vi "Sets the Value for the MX+B Function.vi"(5 "Enable to Query":bool=TRUE, 7 "Enable to Sets":bool=TRUE, 8 "error in":errorcluster, 9 "Offset Factor B":dbl, 10 "Scale Factor M":dbl, 11 "VISA resource name":refnum<visa-resource-name>) -> (0 "error out":errorcluster, 1 "Return the Offset Factor B":string, 2 "Return the Scale Factor M":string, 3 "VISA resource name out":refnum<visa-resource-name>)   [LabVIEW 2011, in "DMM4.lvlib"]
uses:
  <instrlib>/DMM4/DMM4.lvlib
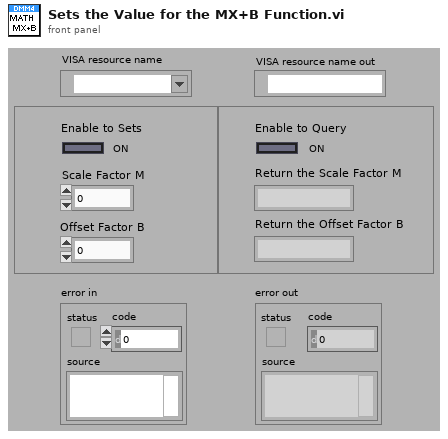
[diagram p1: front panel]
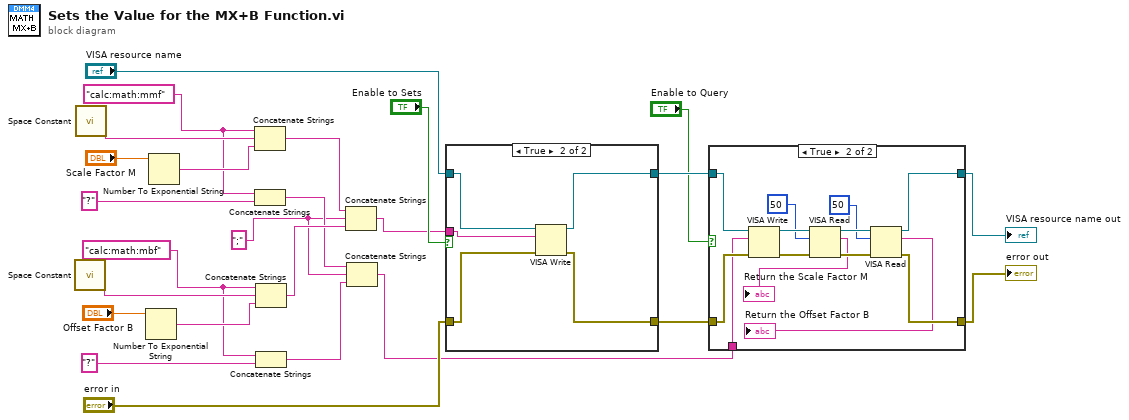
[diagram p0: block diagram]
diagram:
  w12 = ";"
  w16 = "calc:math:mbf"
  w17 = "calc:math:mmf"
  n1 = call <vilib>:"Space Constant.vi"() -> ("String"=w20:string)
  n2 = call <vilib>:"Space Constant.vi"() -> ("String"=w22:string)
  n3 = Number To Exponential String(number="Offset Factor B") -> (E-format string=w21:string)  [unwired: 3 in]
  n4 = Number To Exponential String(number="Scale Factor M") -> (E-format string=w23:string)  [unwired: 3 in]
  n5 = Concatenate Strings(w17, w22, w23) -> (w15:string)
  n6 = Concatenate Strings(w17, "?") -> (w13:string)
  n7 = Concatenate Strings(w16, w20, w21) -> (w14:string)
  n8 = Concatenate Strings(w16, "?") -> (w11:string)
  n9 = Concatenate Strings(w15, w12, w14) -> (w7:string)
  n10 = Concatenate Strings(w13, w12, w11) -> (w1:string)
  n11 = case shown="True" "Enable to Sets" {
    tunnel: "VISA resource name" -> [w27 w32]
    tunnel: "error in" -> [w26 w31]
    tunnel: [w27 w30] -> w6
    tunnel: [w26 w29] -> w5
    tunnel: w7 -> [_ w28]
    frame False {
    }
    frame True {
      n12 = VISA Write(VISA resource name=w32, write buffer=w28, error in (no error)=w31) -> (VISA resource name out=w30:refnum<visa-resource-name>, error out=w29:errorcluster)  [unwired: 1 out]
    }
  }
  n13 = case shown="True" "Enable to Query" {
    tunnel: w6 -> [w34 w41]
    tunnel: w5 -> [w33 w40]
    tunnel: [w34 w39] -> w4
    tunnel: [w33 w38] -> w3
    tunnel: w1 -> [_ w35]
    frame False {
    }
    frame True {
      n14 = VISA Write(VISA resource name=w41, write buffer=w35, error in (no error)=w40) -> (VISA resource name out=w46:refnum<visa-resource-name>, error out=w47:errorcluster)  [unwired: 1 out]
      n15 = VISA Read(VISA resource name=w46, byte count=u32 50, error in (no error)=w47) -> (VISA resource name out=w43:refnum<visa-resource-name>, read buffer=→"Return the Scale Factor M":string, error out=w44:errorcluster)  [unwired: 1 out]
      n16 = VISA Read(VISA resource name=w43, byte count=u32 50, error in (no error)=w44) -> (VISA resource name out=w39:refnum<visa-resource-name>, read buffer=→"Return the Offset Factor B":string, error out=w38:errorcluster)  [unwired: 1 out]
    }
  }
  "VISA resource name out" <- w4
  "error out" <- w3
